vi "Do.vi"(8 "error in (no error)":errorcluster, 10 "Actor in":refnum<class "Actor.lvclass">, 11 "Start Scan Msg":refnum<class "Start Scan Msg.lvclass">) -> (0 "error out":errorcluster, 2 "Actor out":refnum<class "Actor.lvclass">)   [LabVIEW 2016, in "CS++MCS.lvlib" / "Start Scan Msg.lvclass"]
doc: "This VI delivers the message to the actor by calling the appropriate method(s) on the actor."
uses:
  Start Scan Msg.lvclass
  <vilib>/ActorFramework/Actor/Actor.lvclass
  C:/User/Brand/LVP/CSPP-Dev/Packages/CSPP_Core/Actors/CS++PVMonitor Messages/CS++PVUpdate Msg/CS++PVUpdate Msg.lvclass
  CS++MCS/CS++MCS.lvclass
  C:/Program Files (x86)/National Instruments/LabVIEW 2016/vi.lib/ActorFramework/Actor/Actor.lvclass
  CSPP_Core/Actors/CS++PVMonitor Messages/CS++PVUpdate Msg/CS++PVUpdate Msg.lvclass/CS++PVUpdate Msg.ctl
  CSPP_Core/Classes/CS++ProcessVariables/ProcessVariable/PV.lvclass/PV.ctl
  Start Scan Msg.lvclass/Start Scan Msg.ctl
  CSPP_Core/Classes/CS++ProcessVariables/ProcessVariable/PV.lvclass
  CSPP_Core/Actors/CS++PVMonitor Messages/CS++PVUpdate Msg/CS++PVUpdate Msg.lvclass
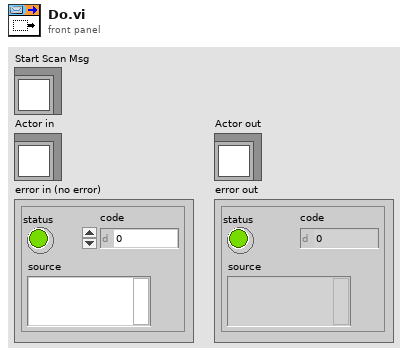
[diagram p1: front panel]
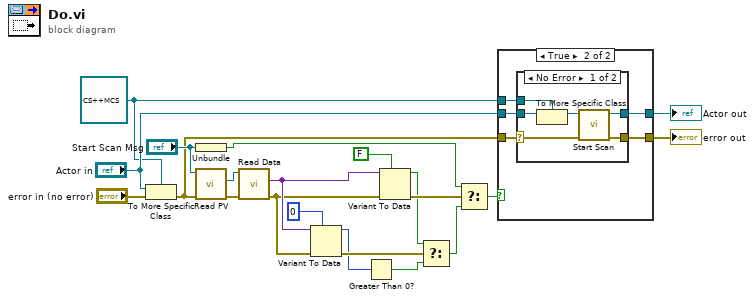
[diagram p0: block diagram]
diagram:
  w17 = refnum<class "CS++MCS.lvclass"> refnum ("Actor in")
  n1 = To More Specific Class(target class=w17, reference="Actor in", error in="error in (no error)") -> (error out=w5:errorcluster)  [unwired: 1 out]
  n2 = Unbundle ("Pre-Unbundler")("Start Scan Msg") -> (w1:bool)
  n3 = call "Read PV.vi"("error in (no error)"=w5, "CS++PVUpdate Msg in"="Start Scan Msg") -> ("error out"=w16:errorcluster, "PV"=w13:refnum<class "PV.lvclass">)  [unwired: 7 in, 1 out]
  n4 = call "Read Data.vi"("error in (no error)"=w16, "PV in"=w13) -> ("error out"=w10:errorcluster, "Data"=w11:variant)  [unwired: 7 in, 1 out]
  n5 = Variant To Data ("I16-Conversion")(error in=w10, type=i16 0 ("I16-Conversion-Constant"), Variant=w11) -> (data=w4:i16, error out=w9:errorcluster)
  n6 = Greater Than 0? ("I16-Comp0")(x=w4) -> (x > 0?=w3:bool)
  n7 = Variant To Data(error in=w10, type=FALSE, Variant=w11) -> (data=w8:bool, error out=w15:errorcluster)
  n8 = Select ("I16-Select")(t=w8, s=w9, f=w3) -> (s? t:f=w7:bool)
  n9 = Select ("MainSelect")(t=w1, s=w15, f=w7) -> (s? t:f=w2:bool)
  n10 = case "Execute?" shown="True" w2 {
    tunnel: [w22 w28] -> w20
    tunnel: [w23 w27] -> w19
    tunnel: "Actor in" -> [w23 w26]
    tunnel: w17 -> [_ w25]
    tunnel: w5 -> [w22 w24]
    frame False {
    }
    frame True {
      n11 = case shown="No Error" w24 {
        selector: w24 -> [w32 w36]
        tunnel: [w34 w36] -> w28
        tunnel: [w33 w35] -> w27
        tunnel: w26 -> [w31 w35]
        tunnel: w25 -> [w30 _]
        frame No Error {
          n12 = To More Specific Class(target class=w30, reference=w31) -> (specific class reference=w29:refnum<class "CS++MCS.lvclass">)  [unwired: 1 in, 1 out]
          n13 = call "Start Scan.vi"("error in (no error)"=w32, "CS++MCS in"=w29) -> ("error out"=w34:errorcluster, "CS++MCS out"=w33:refnum<class "CS++MCS.lvclass">)  [unwired: 8 in]
        }
        frame Error {
        }
      }
    }
  }
  "error out" <- w20
  "Actor out" <- w19
